vi "Write Needed Number.vi"(8 "error in (no error)":errorcluster, 10 "Needed Number":u32, 11 "AverageCollector1D in":refnum<class "AverageCollector1D.lvclass">) -> (0 "error out":errorcluster, 3 "AverageCollector1D out":refnum<class "AverageCollector1D.lvclass">)   [LabVIEW 2014]
uses:
  AverageCollector1D.lvclass
  Observable Actor/Observable Actor.lvclass
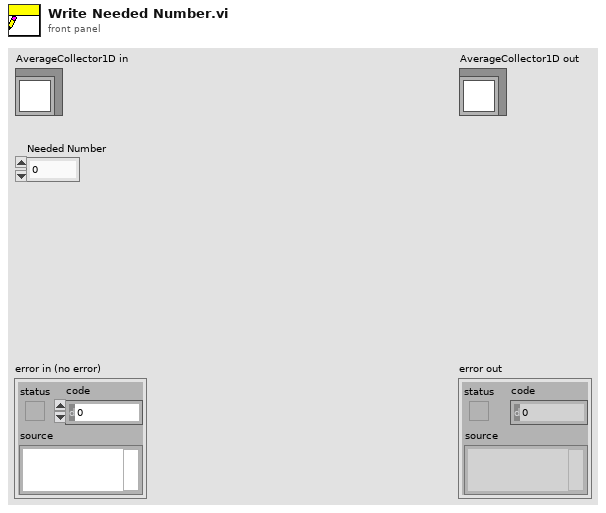
[diagram p1: front panel]
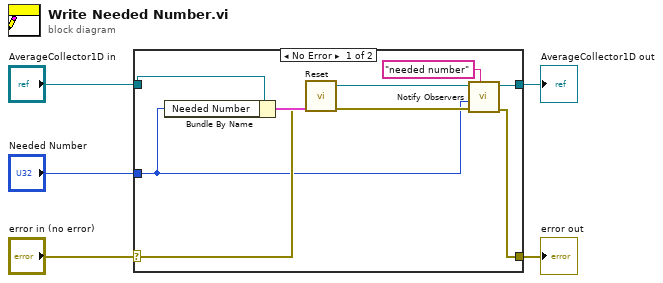
[diagram p0: block diagram]
diagram:
  n1 = case shown="No Error" "error in (no error)" {
    selector: "error in (no error)" -> [w12 w15]
    tunnel: [w8 w15] -> w4
    tunnel: [w10 w16] -> w2
    tunnel: "AverageCollector1D in" -> [w14 w16]
    tunnel: "Needed Number" -> [w7 _]
    frame No Error {
      n2 = Bundle By Name(cluster=w14, "Needed Number"=w7) -> (w13:cluster{})
      n3 = call-dynamic "Reset.vi"("error in (no error)"=w12, "AverageCollector1D in"=w13) -> ("error out"=w9:errorcluster, "AverageCollector1D out"=w11:refnum<class "AverageCollector1D.lvclass">)  [unwired: 8 in]
      n4 = call "Notify Observers.vi"("name"="needed number", "error in (no error)"=w9, "value"=w7, "Observable Actor in"=w11) -> ("error out"=w8:errorcluster, "Observable Actor out"=w10:refnum<class "AverageCollector1D.lvclass">)  [unwired: 6 in]
    }
    frame Error {
    }
  }
  "error out" <- w4
  "AverageCollector1D out" <- w2
